vi "Current Limit.vi"(8 "Speed Setpoint Right":dbl, 9 "Speed Setpoint Left":dbl, 10 "Right Current":dbl format="%#_13g", 11 "Left Current":dbl format="%#_13g") -> (1 "Speed  Right":dbl, 2 "Speed  Left":dbl)   [LabVIEW 2015]
uses:
  Framework/Robot Global Data.vi
panel:
  in  "TPS per current difference":dbl=50.0 format="%#_13g"
  in  "Max Current Per Motor":dbl=40.0 format="%#_13g"
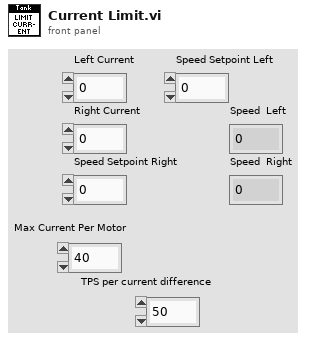
[diagram p1: front panel]
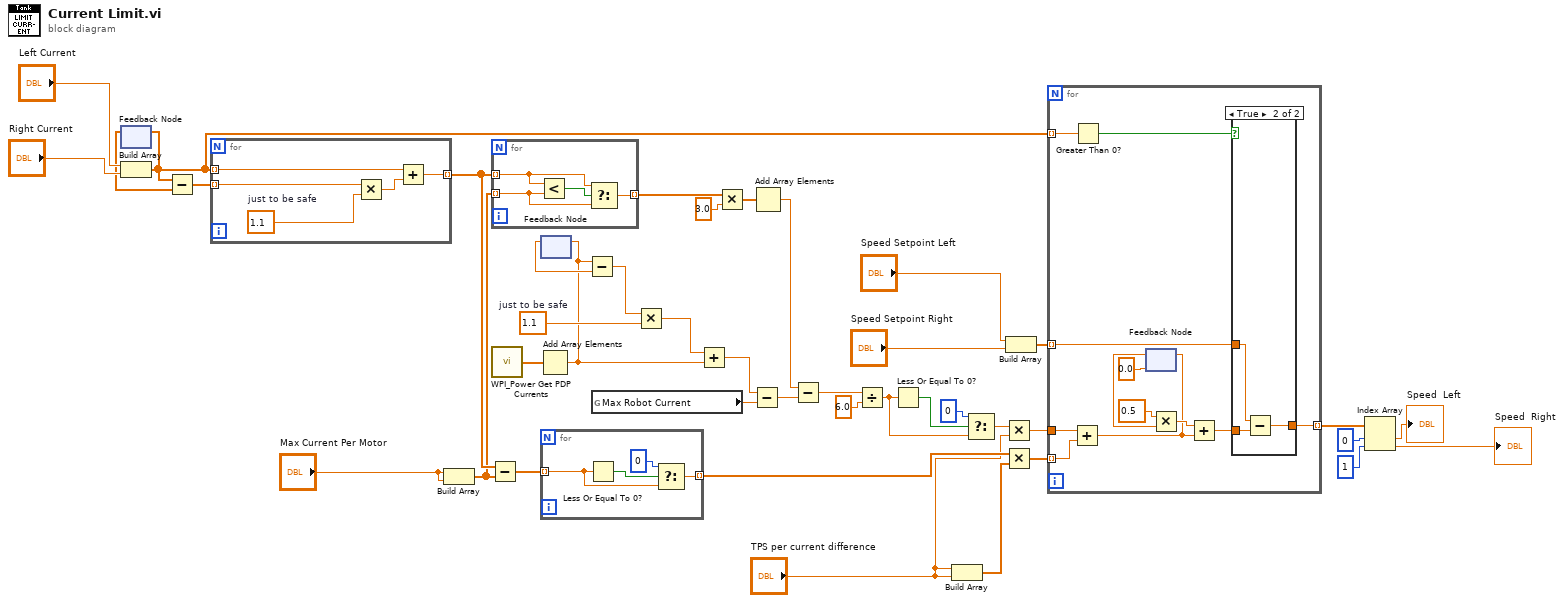
[diagram p0: block diagram]
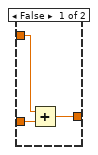
[diagram p2: hidden frame]
diagram:
  w8 = 1.1  # just to be safe
  n1 = feedback #1() -> (w4:dbl[])  [unwired: 1 in]
  n2 = Build Array("Left Current", "Right Current") -> (w3:dbl[])
  n3 = feedback-in #1(w3) -> ()
  n4 = Subtract(x=w3, y=w4) -> (x-y=w41:dbl[])
  n5 = for {
    tunnel: w3 -> [w46] mode=indexing
    tunnel: w41 -> [w44] mode=indexing
    tunnel: [w42] -> w31 mode=indexing
    w43 = 1.1  # just to be safe
    n6 = Multiply(x=w44, y=w43) -> (x*y=w45:dbl)
    n7 = Add(x=w46, y=w45) -> (x+y=w42:dbl)
  }
  n8 = Build Array("Max Current Per Motor", "Max Current Per Motor") -> (w2:dbl[])
  n9 = Subtract(x=w31, y=w2) -> (x-y=w30:dbl[])
  n10 = for {
    tunnel: w31 -> [w49] mode=indexing
    tunnel: w2 -> [w48] mode=indexing
    tunnel: [w47] -> w34 mode=indexing
    n11 = Less?(x=w49, y=w48) -> (x < y?=w50:bool)
    n12 = Select(t=w49, s=w50, f=w48) -> (s? t:f=w47:dbl)
  }
  n13 = call <vilib>:"WPI_Power Get PDP Currents.vi"() -> ("all currents (A)"=w11:dbl[])  [unwired: 13 in, 2 out]
  n14 = Add Array Elements(numeric array=w11) -> (sum=w5:dbl)
  n15 = feedback-in #2(w5) -> ()
  n16 = feedback #2() -> (w10:dbl)  [unwired: 1 in]
  n17 = for {
    tunnel: w30 -> [w52] mode=indexing
    tunnel: [w51] -> w39 mode=indexing
    n18 = Less Or Equal To 0?(x=w52) -> (x <= 0?=w54:bool)
    n19 = Select(t=0, s=w54, f=w52) -> (s? t:f=w51:dbl)
  }
  n20 = Subtract(x=w5, y=w10) -> (x-y=w9:dbl)
  n21 = global read "Robot Global Data.vi" "Max Robot Current"() -> (w12:dbl)
  n22 = Multiply(x=w9, y=w8) -> (x*y=w7:dbl)
  n23 = Add(x=w7, y=w5) -> (x+y=w6:dbl)
  n24 = Multiply(x=w34, y=3.0) -> (x*y=w37:dbl[])
  n25 = Subtract(x=w6, y=w12) -> (x-y=w1:dbl)
  n26 = Add Array Elements(numeric array=w37) -> (sum=w35:dbl)
  n27 = Subtract(x=w35, y=w1) -> (x-y=w33:dbl)
  n28 = Divide(x=w33, y=6.0) -> (x/y=w27:dbl)
  n29 = Less Or Equal To 0?(x=w27) -> (x <= 0?=w29:bool)
  n30 = Build Array("TPS per current difference", "TPS per current difference") -> (w38:dbl[])
  n31 = Select(t=0, s=w29, f=w27) -> (s? t:f=w26:dbl)
  n32 = Multiply(x=w26, y="TPS per current difference") -> (x*y=w23:dbl)
  n33 = Multiply(x=w39, y=w38) -> (x*y=w24:dbl[])
  n34 = Build Array("Speed Setpoint Left", "Speed Setpoint Right") -> (w22:dbl[])
  n35 = for {
    tunnel: w3 -> [w66] mode=indexing
    tunnel: w24 -> [w65] mode=indexing
    tunnel: w23 -> [w64]
    tunnel: w22 -> [w63] mode=indexing
    tunnel: [w62] -> w20 mode=indexing
    n36 = Add(x=w64, y=w65) -> (x+y=w57:dbl)
    n37 = Greater Than 0?(x=w66) -> (x > 0?=w61:bool)
    n38 = feedback-in #3(w57) -> ()
    n39 = feedback #3(0.0) -> (w59:dbl)
    n40 = Multiply(x=0.5, y=w59) -> (x*y=w58:dbl)
    n41 = Add(x=w58, y=w57) -> (x+y=w56:dbl)
    n42 = case shown="True" w61 {
      tunnel: w56 -> [w69 w72]
      tunnel: w63 -> [w68 w71]
      tunnel: [w67 w70] -> w62
      frame False {
        n43 = Add(x=w68, y=w69) -> (x+y=w67:dbl)
      }
      frame True {
        n44 = Subtract(x=w71, y=w72) -> (x-y=w70:dbl)
      }
    }
  }
  n45 = Index Array(array=w20, index #1=0 ("index"), index #2=1 ("index")) -> (element #1=→"Speed  Left":dbl, element #2=→"Speed  Right":dbl)
